vi "ObieHelp.vi"() -> ()   [LabVIEW 2022 SP3]
panel:
  out "Tab Control":enum32{"TOC0", "TOC1"}(tab)
  in  "Table of Contents":i32(listbox)
  in  "OK":bool
  # "Welcome to Oberlin Acoustics version 1\n\nThe Oberlin Acoustics App is an open-source measurement application running on the LabView platform. Versions are available for free for PC and Mac.  \nDeveloped by Chris Rogers and Joseph Curtin. \n\nMany thanks to George Stoppani, for guidence and allowing us to build on his Acquisition and Overlay software.\n\nFeedback is appreciated - please submit it on the website below"
  # "for instructions, help, and troubleshooting,\nplease go to\n\nhttp://sites.google.com/view/oberlinacoustics"
  # "Keyboard Shortcuts"
  # "Zoom a graph:  shift-click on it\nLock cursor to a point: option / ctrl -click and move\nEmail a graph:  shift-click on it\nDelete current position: ESCape key or delete key\nClear entire test: shift-del\nDelete any position: click on the position name in the\n                           banner and select: Delete Position\nMove forward:  space bar\nChange Fading in main plot: use left/right arrow keys - \n                          click multiple times to change fade."
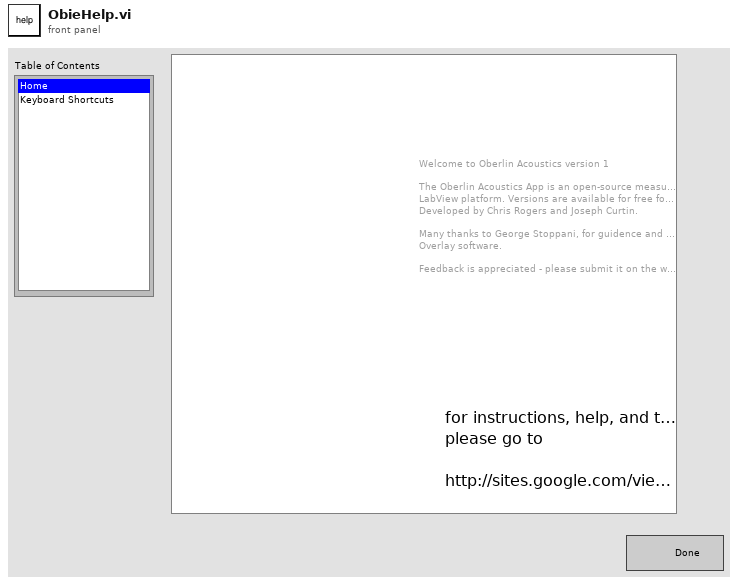
[diagram p1: front panel]
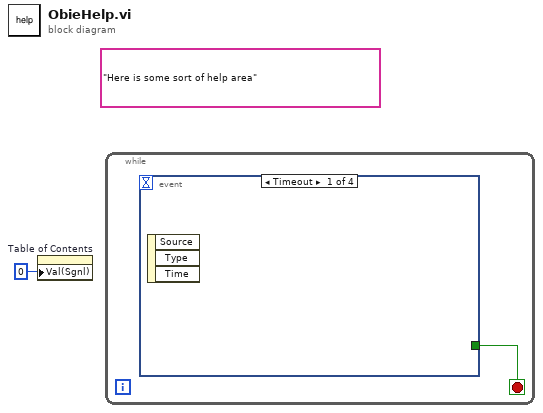
[diagram p0: block diagram]
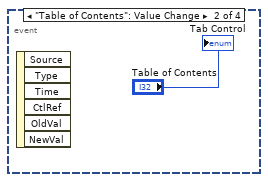
[diagram p2: hidden frame]
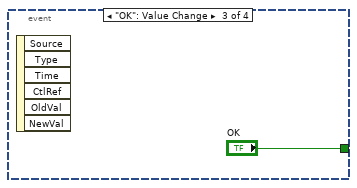
[diagram p3: hidden frame]
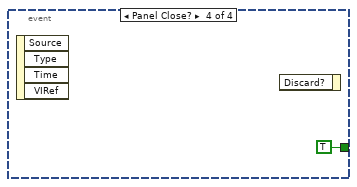
[diagram p4: hidden frame]
diagram:
  (unwired) "Here is some sort of help area" ("URL")
  n1 = property on="Table of Contents" class="LstBox (strict)"("Val(Sgnl)"=0 ("Value (Signaling)")) -> ()  [unwired: 2 in, 2 out]
  n2 = while {
    stop <- w2 stop-if-true
    n3 = event shown="[0] Timeout" {
      selector: _ -> [_ _ _ _]
      dyn-events: _ -> [_ _ _ _]
      timeout: _ -> [_ _ _ _]
      tunnel: [_ _ "OK" TRUE ("OK")] -> w2
      event Timeout {
        n4 = event-data() -> ()  [unwired: 1 in, 3 out]
      }
      event "Table of Contents": Value Change {
        n5 = event-data() -> ()  [unwired: 1 in, 6 out]
        "Tab Control" <- "Table of Contents"
      }
      event "OK": Value Change {
        n6 = event-data() -> ()  [unwired: 1 in, 6 out]
      }
      event Panel Close? {
        n7 = event-data() -> ()  [unwired: 1 in, 4 out]
        n8 = event-data() -> ()  [unwired: 2 in, 1 out]
      }
    }
  }
